vi "SetVolume.vi"(8 "error in (no error)":errorcluster, 11 "Volume":u32) -> (0 "error out":errorcluster)   [LabVIEW 2014, in "LabBASSMOD2.lvlib"]
uses:
  LabBASSMOD2.lvlib
  DLL/BASSMOD.dll
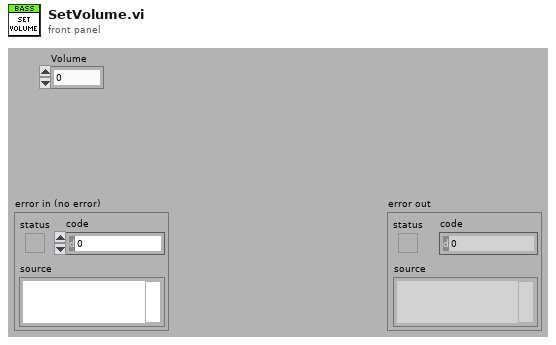
[diagram p1: front panel]
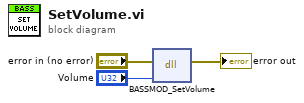
[diagram p0: block diagram]
diagram:
  n1 = dll-call lib="C:/dev/PGS/LabBASSMOD2/DLL/BASSMOD.dll" fn="BASSMOD_SetVolume" ("BASSMOD_MusicStop")(error in="error in (no error)", "volume"="Volume") -> (error out=→"error out":errorcluster)  [unwired: 4 in, 1 out]
